vi "Send.vi"(0 "Ch1":i32, 1 "Ch2":i32, 2 "Ch3":i32, 3 "Ch4":i32, 4 "Ch5":i32, 7 "error in (no error)":errorcluster) -> (20 "function return":bool, 27 "error out":errorcluster)   [LabVIEW 2013, in "PCTx.lvlib"]
doc: "DECLDIR bool Send(int delay1,int delay2,int delay3,int delay4,int delay5,int delay6,int delay7,int delay8,\n int delay9,int delay10,int delay11,int delay12,int delay13,int delay14,int delay15,int delay16,\n int delay17,int delay18,int delay19,int delay20,int delay21,int delay22,int delay23,int delay24,\n int delay25);"
uses:
  PCTx.lvlib
  PCTx.dll
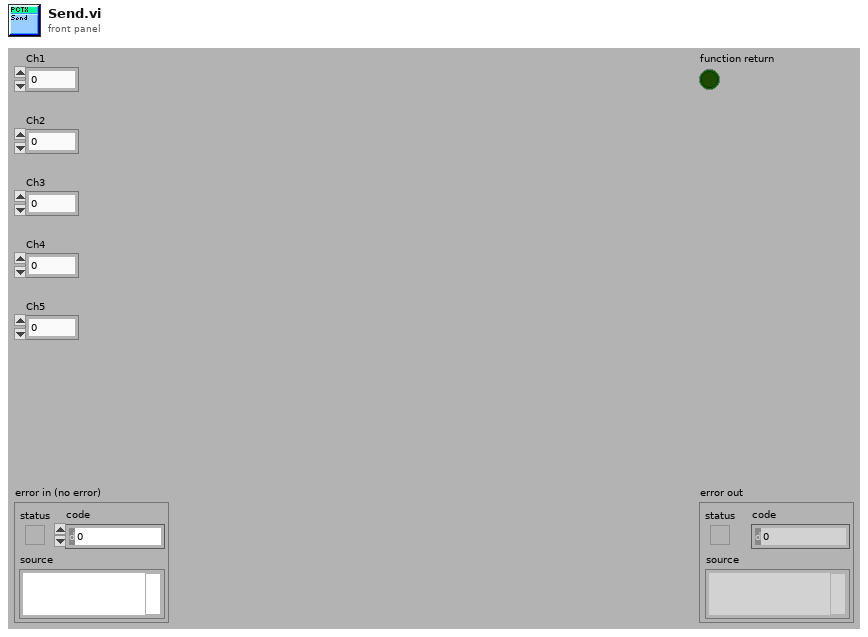
[diagram p1: front panel]
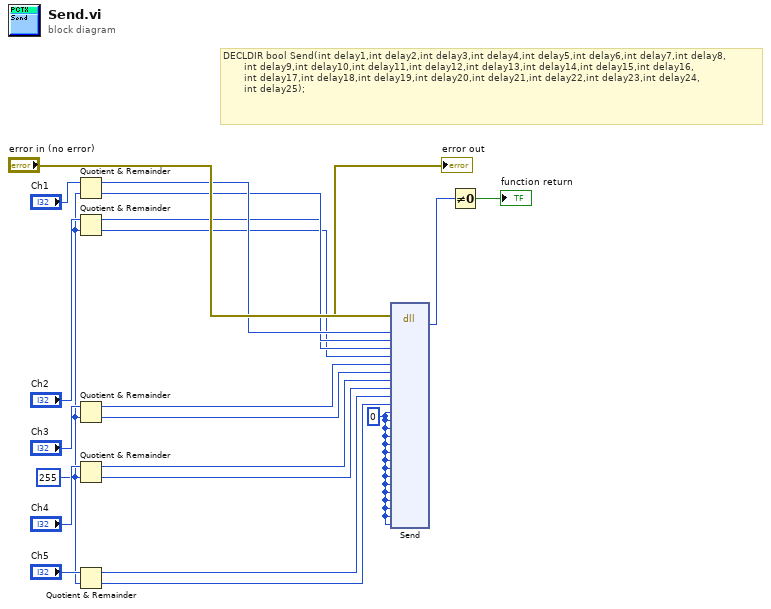
[diagram p0: block diagram]
diagram:
  w11 = 255
  w17 = 0
  # "DECLDIR bool Send(int delay1,int delay2,int delay3,int delay4,int delay5,int delay6,int delay7,int delay8,\n\t\t\t\t\t  int delay9,int delay10,int delay11,int delay12,int delay13,int delay14,int delay15,int delay16,\n\t\t\t\t\t  int delay17,int delay18,int delay19,int delay20,int delay21,int delay22,int delay23,int delay24,\n\t\t\t\t\t  int delay25);"
  n1 = Quotient & Remainder(x="Ch1", y=w11) -> (x-y*floor(x/y)=w10:i32, floor(x/y)=w9:i32)
  n2 = Quotient & Remainder(x="Ch2", y=w11) -> (x-y*floor(x/y)=w8:i32, floor(x/y)=w7:i32)
  n3 = Quotient & Remainder(x="Ch3", y=w11) -> (x-y*floor(x/y)=w6:i32, floor(x/y)=w5:i32)
  n4 = Quotient & Remainder(x="Ch4", y=w11) -> (x-y*floor(x/y)=w4:i32, floor(x/y)=w3:i32)
  n5 = Quotient & Remainder(x="Ch5", y=w11) -> (x-y*floor(x/y)=w2:i32, floor(x/y)=w1:i32)
  n6 = dll-call lib="C:/Users/user/Documents/Dropbox/Kettering/Robotics Team/RC Car Race Information/Teleop Labview Code/Winter '14 Force Feedback Experiment/PCTx Files/PCTx/PCTx.*" fn="Send"(error in="error in (no error)", "delay1"=w10, "delay2"=w9, "delay3"=w8, "delay4"=w7, "delay5"=w6, "delay6"=w5, "delay7"=w4, "delay8"=w3, "delay9"=w2, "delay10"=w1, "delay11"=w17, "delay12"=w17, "delay13"=w17, "delay14"=w17, "delay15"=w17, "delay16"=w17, "delay17"=w17, "delay18"=w17, "delay19"=w17, "delay20"=w17, "delay21"=w17, "delay22"=w17, "delay23"=w17, "delay24"=w17, "delay25"=w17) -> (error out=→"error out":errorcluster, "return type"=w20:u8)  [unwired: 27 in, 1 out]
  n7 = Not Equal To 0?(x=w20) -> (x != 0?=→"function return":bool)
